vi "botted input.vi"(8 "hold note key":T2, 9 "next note":cluster{"1st rail":i32, "2nd rail":i32}, 10 "song info":T3, 11 "progress":dbl) -> (3 "keys pressed":T1(array[ring]))   [LabVIEW 2023]
panel:
  out "x":T1(array[ring])
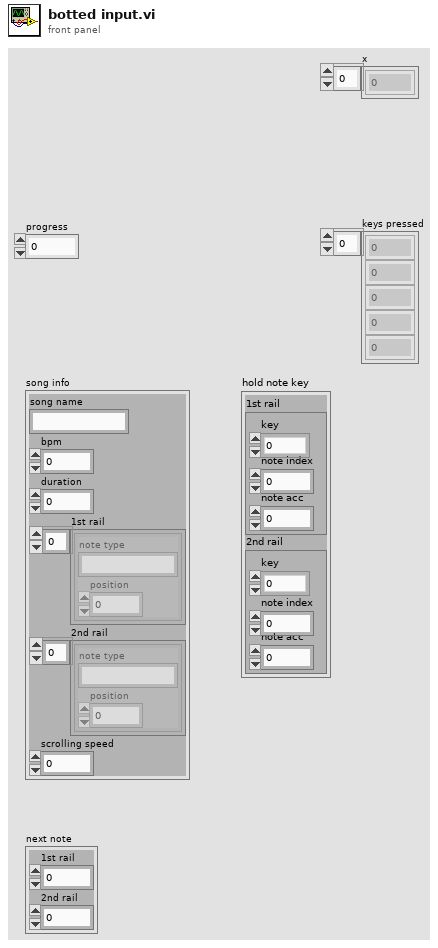
[diagram p1: front panel]
types:
  T1 = enum16{"0", "1", "2", "3", "4", "5", "6", "7", "8", "9", "A", "B", "C", "D", "E", "F", "G", "H", "I", "J", "K", "L", "M", "N", "O", "P", "Q", "R", "S", "T", "U", "V", "W", "X", "Y", "Z", "F1", "F2", "F3", "F4", "F5", "F6", "F7", "F8", "F9", "F10", "F11", "F12", "F13", "F14", "F15", "ADD", "BACK", "BACKSLASH", "CAPITAL", "COMMA", "DECIMAL", "DELETE", "DIVIDE", "DOWN", "END", "EQUALS", "ESCAPE", "GRAVE (`)", "HOME", "INSERT", "LBRACKET", "LCONTROL", "LEFT", "L ALT", "LSHIFT", "LWIN", "MINUS", "MULTIPLY", "NEXT", "NUMLOCK", "NUMPAD_0", "NUMPAD_1", "NUMPAD_2", "NUMPAD_3", "NUMPAD_4", "NUMPAD_5", "NUMPAD_6", "NUMPAD_7", "NUMPAD_8", "NUMPAD_9", "PAUSE", "PERIOD", "PRIOR (PG UP)", "RBRACKET", "RCONTROL", "RETURN", "RIGHT", "R ALT", "RSHIFT", "RWIN", "SCROLL", "SEMICOLON", "SLASH", "SPACE", "SUBTRACT", "TAB", "UP", "ENTER (num pad)", "' (quote)"}[]
  T2 = cluster{"1st rail":cluster{"key":enum16{"0", "1", "2", "3", "4", "5", "6", "7", "8", "9", "A", "B", "C", "D", "E", "F", "G", "H", "I", "J", "K", "L", "M", "N", "O", "P", "Q", "R", "S", "T", "U", "V", "W", "X", "Y", "Z", "F1", "F2", "F3", "F4", "F5", "F6", "F7", "F8", "F9", "F10", "F11", "F12", "F13", "F14", "F15", "ADD", "BACK", "BACKSLASH", "CAPITAL", "COMMA", "DECIMAL", "DELETE", "DIVIDE", "DOWN", "END", "EQUALS", "ESCAPE", "GRAVE (`)", "HOME", "INSERT", "LBRACKET", "LCONTROL", "LEFT", "L ALT", "LSHIFT", "LWIN", "MINUS", "MULTIPLY", "NEXT", "NUMLOCK", "NUMPAD_0", "NUMPAD_1", "NUMPAD_2", "NUMPAD_3", "NUMPAD_4", "NUMPAD_5", "NUMPAD_6", "NUMPAD_7", "NUMPAD_8", "NUMPAD_9", "PAUSE", "PERIOD", "PRIOR (PG UP)", "RBRACKET", "RCONTROL", "RETURN", "RIGHT", "R ALT", "RSHIFT", "RWIN", "SCROLL", "SEMICOLON", "SLASH", "SPACE", "SUBTRACT", "TAB", "UP", "ENTER (num pad)", "' (quote)"}, "note index":i32, "note acc":i32}, "2nd rail":cluster{"key":enum16{"0", "1", "2", "3", "4", "5", "6", "7", "8", "9", "A", "B", "C", "D", "E", "F", "G", "H", "I", "J", "K", "L", "M", "N", "O", "P", "Q", "R", "S", "T", "U", "V", "W", "X", "Y", "Z", "F1", "F2", "F3", "F4", "F5", "F6", "F7", "F8", "F9", "F10", "F11", "F12", "F13", "F14", "F15", "ADD", "BACK", "BACKSLASH", "CAPITAL", "COMMA", "DECIMAL", "DELETE", "DIVIDE", "DOWN", "END", "EQUALS", "ESCAPE", "GRAVE (`)", "HOME", "INSERT", "LBRACKET", "LCONTROL", "LEFT", "L ALT", "LSHIFT", "LWIN", "MINUS", "MULTIPLY", "NEXT", "NUMLOCK", "NUMPAD_0", "NUMPAD_1", "NUMPAD_2", "NUMPAD_3", "NUMPAD_4", "NUMPAD_5", "NUMPAD_6", "NUMPAD_7", "NUMPAD_8", "NUMPAD_9", "PAUSE", "PERIOD", "PRIOR (PG UP)", "RBRACKET", "RCONTROL", "RETURN", "RIGHT", "R ALT", "RSHIFT", "RWIN", "SCROLL", "SEMICOLON", "SLASH", "SPACE", "SUBTRACT", "TAB", "UP", "ENTER (num pad)", "' (quote)"}, "note index":i32, "note acc":i32}}
  T3 = cluster{"song name":string, "bpm":i32, "duration":i32, "1st rail":cluster{"note type":string, "position":dbl}[], "2nd rail":cluster{"note type":string, "position":dbl}[], "scrolling speed":dbl}
  T4 = enum16{"0", "1", "2", "3", "4", "5", "6", "7", "8", "9", "A", "B", "C", "D", "E", "F", "G", "H", "I", "J", "K", "L", "M", "N", "O", "P", "Q", "R", "S", "T", "U", "V", "W", "X", "Y", "Z", "F1", "F2", "F3", "F4", "F5", "F6", "F7", "F8", "F9", "F10", "F11", "F12", "F13", "F14", "F15", "ADD", "BACK", "BACKSLASH", "CAPITAL", "COMMA", "DECIMAL", "DELETE", "DIVIDE", "DOWN", "END", "EQUALS", "ESCAPE", "GRAVE (`)", "HOME", "INSERT", "LBRACKET", "LCONTROL", "LEFT", "L ALT", "LSHIFT", "LWIN", "MINUS", "MULTIPLY", "NEXT", "NUMLOCK", "NUMPAD_0", "NUMPAD_1", "NUMPAD_2", "NUMPAD_3", "NUMPAD_4", "NUMPAD_5", "NUMPAD_6", "NUMPAD_7", "NUMPAD_8", "NUMPAD_9", "PAUSE", "PERIOD", "PRIOR (PG UP)", "RBRACKET", "RCONTROL", "RETURN", "RIGHT", "R ALT", "RSHIFT", "RWIN", "SCROLL", "SEMICOLON", "SLASH", "SPACE", "SUBTRACT", "TAB", "UP", "ENTER (num pad)", "' (quote)"}
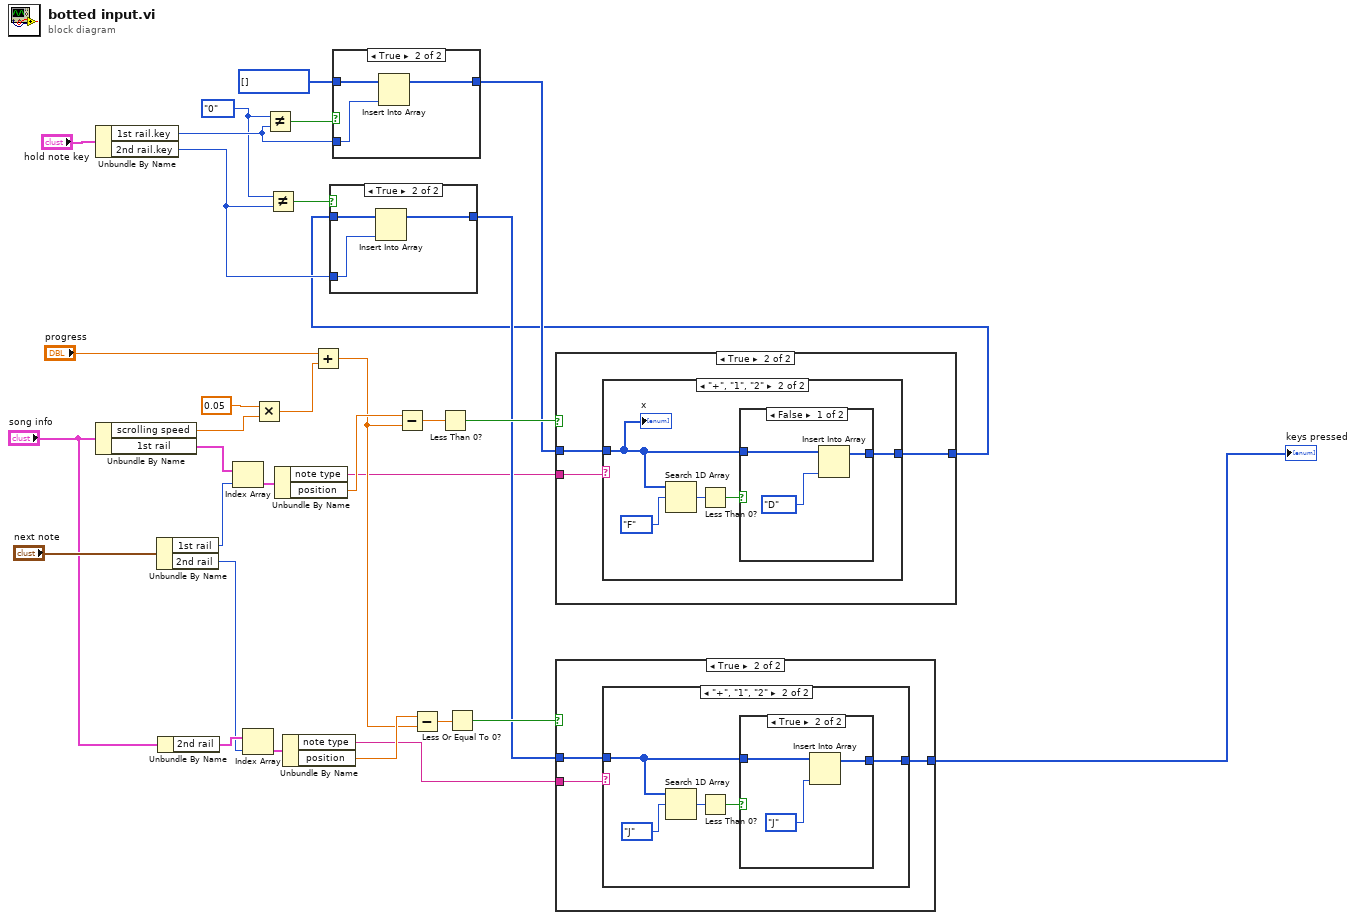
[diagram p0: block diagram]
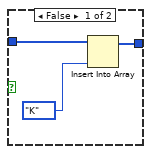
[diagram p5: hidden frame]
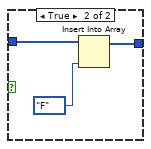
[diagram p9: hidden frame]
diagram:
  w11 = T1 [] items=["0", "1", "2", "3", "4", "5", "6", "7", "8", "9", "A", "B", "C", "D", "E", "F", "G", "H", "I", "J", "K", "L", "M", "N", "O", "P", "Q", "R", "S", "T", "U", "V", "W", "X", "Y", "Z", "F1", "F2", "F3", "F4", "F5", "F6", "F7", "F8", "F9", "F10", "F11", "F12", "F13", "F14", "F15", "ADD", "BACK", "BACKSLASH", "CAPITAL", "COMMA", "DECIMAL", "DELETE", "DIVIDE", "DOWN", "END", "EQUALS", "ESCAPE", "GRAVE (`)", "HOME", "INSERT", "LBRACKET", "LCONTROL", "LEFT", "L ALT", "LSHIFT", "LWIN", "MINUS", "MULTIPLY", "NEXT", "NUMLOCK", "NUMPAD_0", "NUMPAD_1", "NUMPAD_2", "NUMPAD_3", "NUMPAD_4", "NUMPAD_5", "NUMPAD_6", "NUMPAD_7", "NUMPAD_8", "NUMPAD_9", "PAUSE", "PERIOD", "PRIOR (PG UP)", "RBRACKET", "RCONTROL", "RETURN", "RIGHT", "R ALT", "RSHIFT", "RWIN", "SCROLL", "SEMICOLON", "SLASH", "SPACE", "SUBTRACT", "TAB", "UP", "ENTER (num pad)", "' (quote)"] ("x")
  w13 = T4."0" ("x")
  n1 = Unbundle By Name("hold note key") -> ("1st rail.key"=w23:T4, "2nd rail.key"=w10:T4)
  n2 = Unbundle By Name("song info") -> ("scrolling speed"=w5:dbl, "1st rail"=w31:cluster{"note type":string, "position":dbl}[])
  n3 = Unbundle By Name("next note") -> ("1st rail"=w30:i32, "2nd rail"=w19:i32)
  n4 = Unbundle By Name("song info") -> ("2nd rail"=w20:cluster{"note type":string, "position":dbl}[])
  n5 = Index Array(array=w31, index=w30) -> (element=w29:cluster{"note type":string, "position":dbl})
  n6 = Index Array(array=w20, index=w19) -> (element=w18:cluster{"note type":string, "position":dbl})
  n7 = Multiply(x=0.05, y=w5) -> (x*y=w3:dbl)
  n8 = Not Equal?(x=w13, y=w23) -> (x != y?=w24:bool)
  n9 = Not Equal?(x=w13, y=w10) -> (x != y?=w12:bool)
  n10 = Unbundle By Name(w29) -> ("note type"=w1:string, "position"=w28:dbl)
  n11 = Unbundle By Name(w18) -> ("note type"=w14:string, "position"=w17:dbl)
  n12 = Add(x="progress", y=w3) -> (x+y=w6:dbl)
  n13 = case shown="True" w24 {
    tunnel: w23 -> [_ w36]
    tunnel: w11 -> [w33 w35]
    tunnel: [w33 w34] -> w22
    frame False {
    }
    frame True {
      n14 = Insert Into Array(array=w35, new element=w36) -> (w34:T1)  [unwired: 1 in]
    }
  }
  n15 = Subtract(x=w28, y=w6) -> (x-y=w27:dbl)
  n16 = Subtract(x=w17, y=w6) -> (x-y=w16:dbl)
  n17 = Less Than 0?(x=w27) -> (x < 0?=w26:bool)
  n18 = Less Or Equal To 0?(x=w16) -> (x <= 0?=w15:bool)
  n19 = case shown="True" w26 {
    tunnel: w1 -> [_ w40]
    tunnel: w22 -> [w37 w39]
    tunnel: [w37 w38] -> w2
    frame False {
    }
    frame True {
      n20 = case shown="\"+\", \"1\", \"2\"" w40 {
        tunnel: w39 -> [w41 w42]
        tunnel: [w41 w43] -> w38
        frame Default {
        }
        frame "+", "1", "2" {
          n21 = Search 1D Array(1D array=w42, element=T4."F" ("x")) -> (index of element=w45:i32)  [unwired: 1 in]
          n22 = Less Than 0?(x=w45) -> (x < 0?=w44:bool)
          n23 = case shown="False" w44 {
            tunnel: w42 -> [w49 w51]
            tunnel: [w48 w50] -> w43
            frame False {
              n24 = Insert Into Array(array=w49, new element=T4."D" ("x")) -> (w48:T1)  [unwired: 1 in]
            }
            frame True {
              n25 = Insert Into Array(array=w51, new element=T4."F" ("x")) -> (w50:T1)  [unwired: 1 in]
            }
          }
          "x" <- w42
        }
      }
    }
  }
  n26 = case shown="True" w12 {
    tunnel: w10 -> [_ w56]
    tunnel: w2 -> [w53 w55]
    tunnel: [w53 w54] -> w9
    frame False {
    }
    frame True {
      n27 = Insert Into Array(array=w55, new element=w56) -> (w54:T1)  [unwired: 1 in]
    }
  }
  n28 = case shown="True" w15 {
    tunnel: w14 -> [_ w60]
    tunnel: w9 -> [w57 w59]
    tunnel: [w57 w58] -> w8
    frame False {
    }
    frame True {
      n29 = case shown="\"+\", \"1\", \"2\"" w60 {
        tunnel: w59 -> [w61 w64]
        tunnel: [w61 w62] -> w58
        frame Default {
        }
        frame "+", "1", "2" {
          n30 = Search 1D Array(1D array=w64, element=T4."J" ("x")) -> (index of element=w65:i32)  [unwired: 1 in]
          n31 = Less Than 0?(x=w65) -> (x < 0?=w63:bool)
          n32 = case shown="True" w63 {
            tunnel: w64 -> [w69 w71]
            tunnel: [w68 w70] -> w62
            frame False {
              n33 = Insert Into Array(array=w69, new element=T4."K" ("x")) -> (w68:T1)  [unwired: 1 in]
            }
            frame True {
              n34 = Insert Into Array(array=w71, new element=T4."J" ("x")) -> (w70:T1)  [unwired: 1 in]
            }
          }
        }
      }
    }
  }
  "keys pressed" <- w8
